vi "Add Digital Input Channels.vi"(8 "error in (no error)":errorcluster, 9 "DIO Port Settings":T1[](array[typedef]), 11 "DAQ Ref":refnum<k24>) -> (0 "error out":errorcluster, 3 "DAQ Ref":refnum<k24>)   [LabVIEW 2019, in "Simple SysDef API.lvlib"]
uses:
  <userlib>/SimpleSysDef/Simple SysDef API.lvlib
  NationalInstruments.VeriStand.SystemDefinitionAPI
  <userlib>/SimpleSysDef/_SubVIs/Add DAQ Hardware_Digital Port Settings.ctl
  <userlib>/SimpleSysDef/_SubVIs/Add DAQ Hardware_Digital Settings.ctl
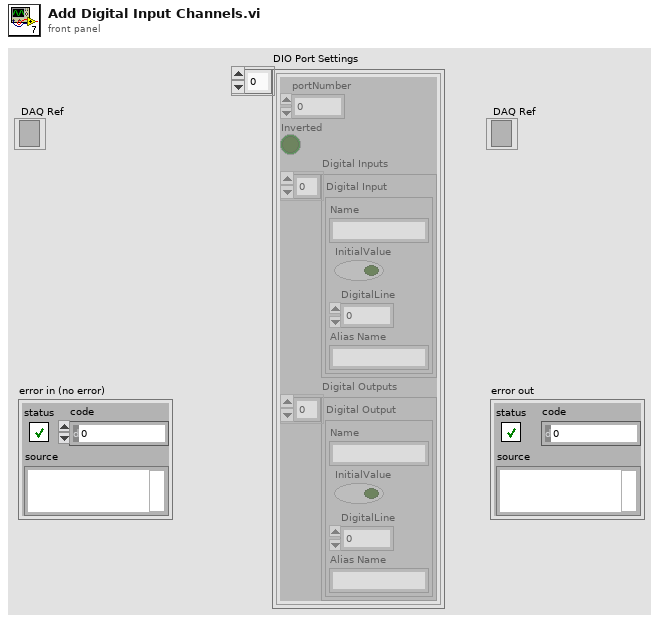
[diagram p1: front panel]
types:
  T1 = typedef "Simple SysDef API.lvlib/Add DAQ Hardware_Digital Port Settings.ctl" = cluster{"portNumber":u32, "Inverted":bool, "Digital Inputs":T2[], "Digital Outputs":T2[]}
  T2 = typedef "Simple SysDef API.lvlib/Add DAQ Hardware_Digital Settings.ctl" = cluster{"Name":string, "InitialValue":bool, "DigitalLine":u32, "Alias Name":string}
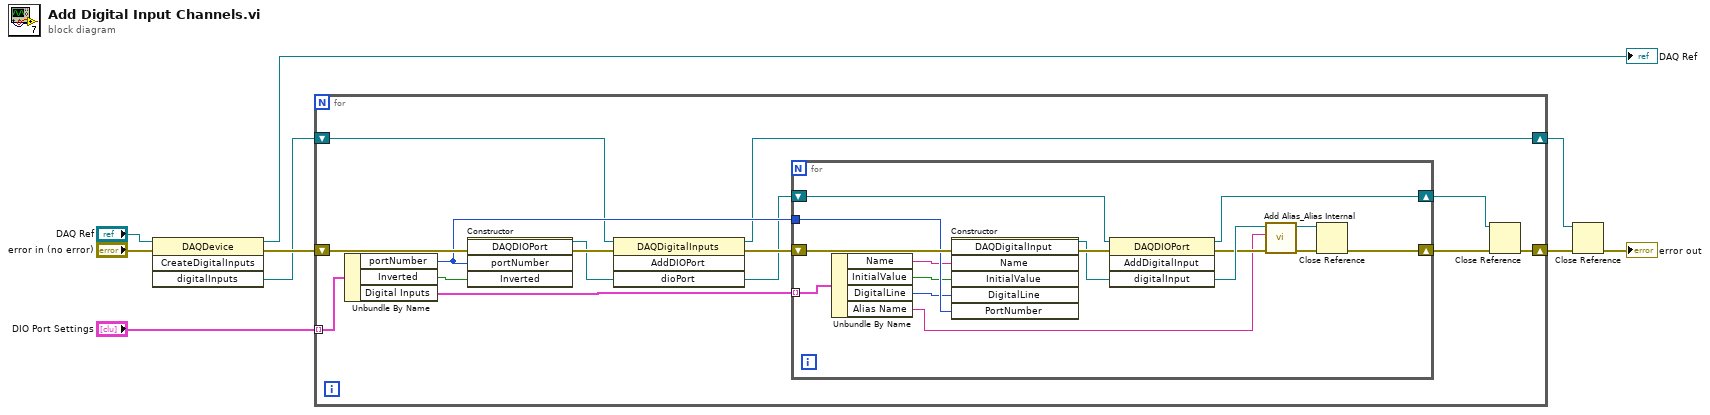
[diagram p0: block diagram]
diagram:
  n1 = invoke class="DAQDevice" method="CreateDigitalInputs"(reference="DAQ Ref", error in="error in (no error)") -> (reference out=→"DAQ Ref":refnum<k24>, error out=w4:errorcluster, "digitalInputs"=w1:refnum<k24>)  [unwired: 2 in, 1 out]
  n2 = for {
    shift-right: [w21] -> w6
    shift-left: w4 -> [w22]
    shift-right: [w11] -> w7
    shift-left: w1 -> [w12]
    tunnel: "DIO Port Settings" -> [w18] mode=indexing
    n3 = Unbundle By Name(w18) -> ("portNumber"=w19:u32, "Inverted"=w20:bool, "Digital Inputs"=w17:T2[])
    n4 = constructor class="DAQDIOPort"(error in=w22, "portNumber"=w19, "Inverted"=w20) -> (reference out=w10:refnum<k24>, error out=w14:errorcluster)  [unwired: 2 in, 3 out]
    n5 = invoke class="DAQDigitalInputs" method="AddDIOPort"(reference=w12, error in=w14, "dioPort"=w10) -> (reference out=w11:refnum<k24>, error out=w13:errorcluster)  [unwired: 1 in, 2 out]
    n6 = for {
      shift-right: [w33] -> w15
      shift-left: w13 -> [w35]
      shift-right: [w36] -> w16
      shift-left: w10 -> [w37]
      tunnel: w19 -> [w32]
      tunnel: w17 -> [w31] mode=indexing
      n7 = Unbundle By Name(w31) -> ("Name"=w28:string, "InitialValue"=w29:bool, "DigitalLine"=w30:u32, "Alias Name"=w23:string)
      n8 = constructor class="DAQDigitalInput"(error in=w35, "Name"=w28, "InitialValue"=w29, "DigitalLine"=w30, "PortNumber"=w32) -> (reference out=w27:refnum<k24>, error out=w34:errorcluster)  [unwired: 2 in, 5 out]
      n9 = invoke class="DAQDIOPort" method="AddDigitalInput"(reference=w37, error in=w34, "digitalInput"=w27) -> (reference out=w36:refnum<k24>, error out=w25:errorcluster)  [unwired: 1 in, 2 out]
      n10 = call <userlib>:"Add Alias_Alias Internal.vi"("error in (no error)"=w25, "Name"=w23, "Base Node"=w27) -> ("error out"=w24:errorcluster, "Base Node out"=w26:refnum<k24>)  [unwired: 7 in]
      n11 = Close Reference(reference=w26, error in (no error)=w24) -> (error out=w33:errorcluster)
    }
    n12 = Close Reference(reference=w16, error in (no error)=w15) -> (error out=w21:errorcluster)
  }
  n13 = Close Reference(reference=w7, error in (no error)=w6) -> (error out=→"error out":errorcluster)
